vi "TagDB Refmgr-Execute Expression.vi"(8 "error in (no error)":errorcluster, 10 "expressions":cluster{"Tag":string, "formula":string}[](array[cluster]), 11 "DB Ref":T1) -> (0 "error out":errorcluster, 1 "time(ms)":u32, 3 "DB Ref (dup)":T1)   [LabVIEW 2017, in "TagDB UIStateExpression.lvlib"]
uses:
  TagDB UIStateExpression.lvlib
  <userlib>/_NEVSTOP/TagDB/Typedef/TagDB.ctl
  <userlib>/_OpenG.lib/string/string.llb/Trim Whitespace (String)__ogtk.vi
  <userlib>/_OpenG.lib/string/string.llb/Trim Whitespace (String Array)__ogtk.vi
  <userlib>/_OpenG.lib/array/array.llb/Filter 1D Array with Scalar (String)__ogtk.vi
  <userlib>/_NEVSTOP/TagDB/TagDB.lvlib
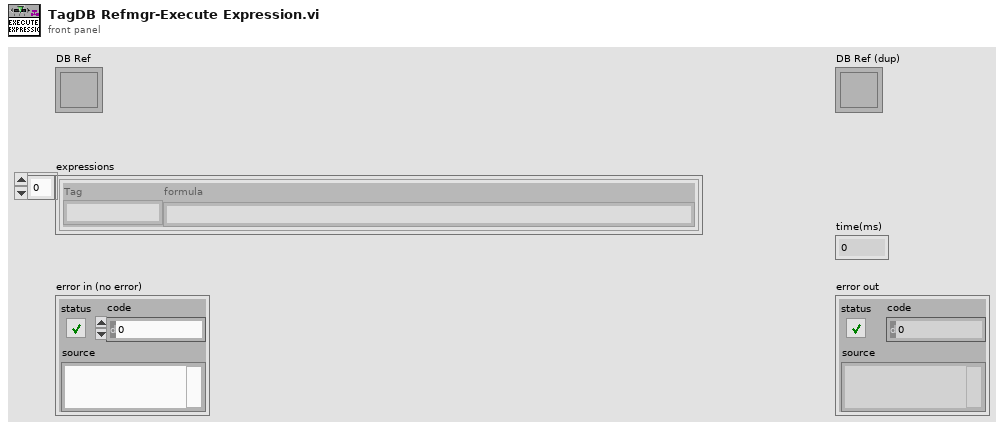
[diagram p1: front panel]
types:
  T1 = typedef "TagDB.lvlib/TagDB.ctl" = refnum<k1>
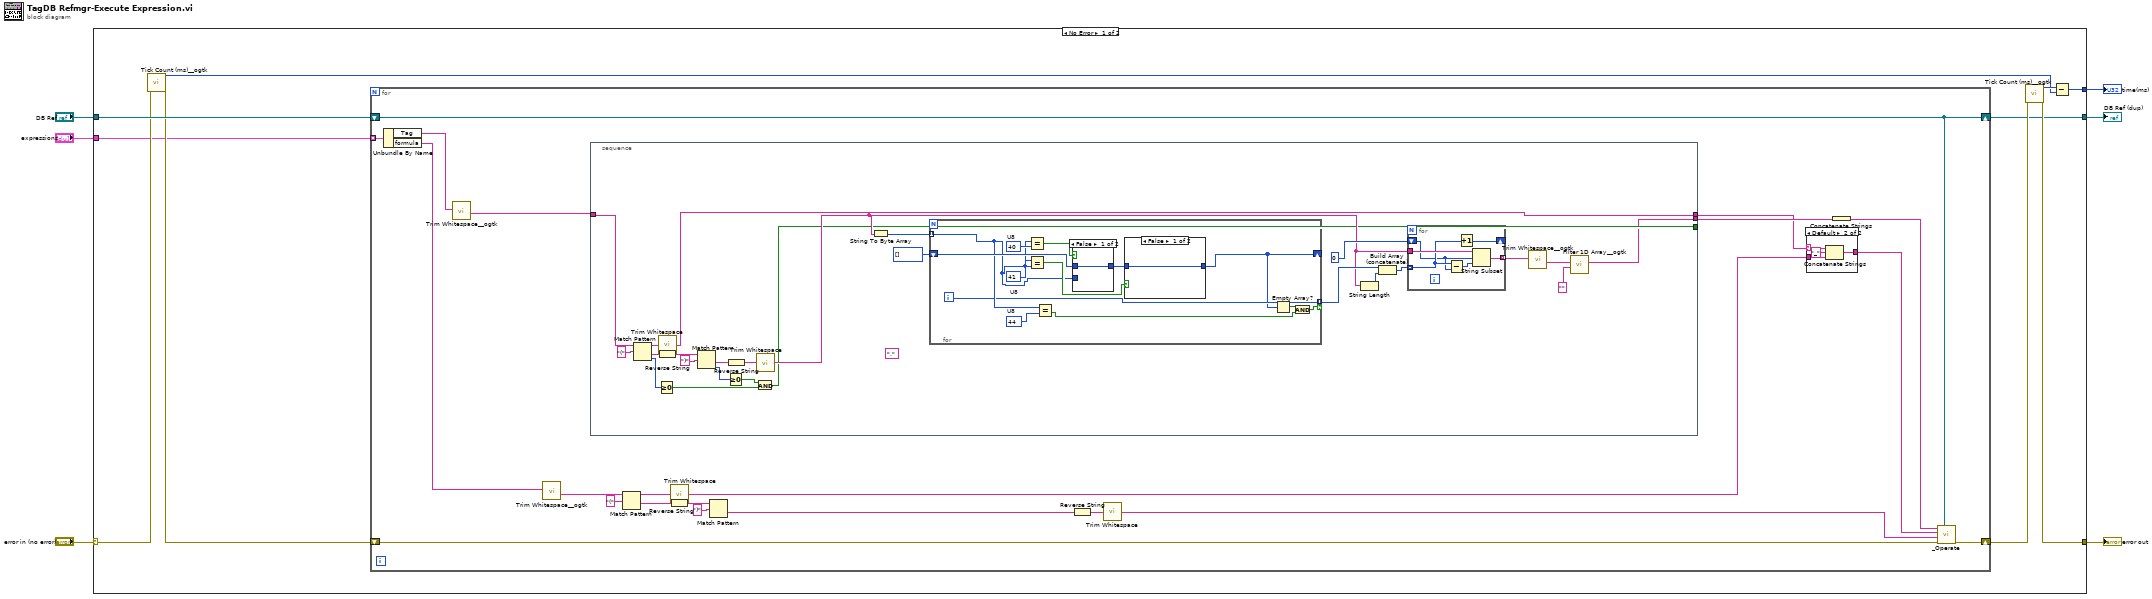
[diagram p0: block diagram]
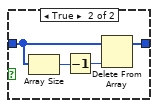
[diagram p2: hidden frame]
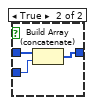
[diagram p3: hidden frame]
diagram:
  n1 = case shown="No Error" "error in (no error)" {
    selector: "error in (no error)" -> [w15 w97]
    tunnel: [w12 w97] -> w5
    tunnel: "DB Ref" -> [w16 w96]
    tunnel: [w8 w96] -> w1
    tunnel: [w9 _] -> w3
    tunnel: "expressions" -> [w7 _]
    frame No Error {
      n2 = call <userlib>:"Tick Count (ms)__ogtk.vi"("error in (no error)"=w15) -> ("error out"=w13:errorcluster, "millisecond timer value"=w10:u32)  [unwired: 9 in]
      n3 = for {
        tunnel: w7 -> [w37] mode=indexing
        shift-right: [w35] -> w14
        shift-left: w13 -> [w36]
        shift-right: [w34] -> w8
        shift-left: w16 -> [w34]
        n4 = Unbundle By Name(w37) -> ("Tag"=w33:string, "formula"=w32:string)
        n5 = call-poly <userlib>:"Trim Whitespace__ogtk.vi"("String in"=w33) -> ("String out"=w31:string)  [unwired: 6 in]
        n6 = call-poly <userlib>:"Trim Whitespace__ogtk.vi"("String in"=w32) -> ("String out"=w21:string)  [unwired: 6 in]
        n7 = stacked-sequence {
          tunnel: [w48] -> _
          tunnel: [w43] -> w30
          tunnel: [w52] -> w29
          tunnel: w31 -> [w40]
          frame #0 {
            (unwired) "," ("regular expression")
            n8 = Match Pattern(string=w40, regular expression="(") -> (before substring=w39:string, after substring=w41:string, offset past match=w44:i32)  [unwired: 1 in, 1 out]
            n9 = Greater Or Equal To 0?(x=w44) -> (x >= 0?=w47:bool)
            n10 = call <vilib>:"Trim Whitespace.vi"("string"=w39) -> ("trimmed string"=w52:string)  [unwired: 1 in]
            n11 = Reverse String(1:w41) -> (0:w49:string)
            n12 = Match Pattern(string=w49, regular expression=")") -> (after substring=w50:string, offset past match=w45:i32)  [unwired: 1 in, 2 out]
            n13 = Greater Or Equal To 0?(x=w45) -> (x >= 0?=w46:bool)
            n14 = Reverse String(1:w50) -> (0:w51:string)
            n15 = And(x=w46, y=w47) -> (x .and. y?=w48:bool)
            n16 = call <vilib>:"Trim Whitespace.vi"("string"=w51) -> ("trimmed string"=w53:string)  [unwired: 1 in]
            n17 = String To Byte Array(string=w53) -> (unsigned byte array=w55:u8[])
            n18 = for {
              tunnel: w55 -> [w74] mode=indexing
              shift-right: [w71] -> _
              shift-left: i32[] [] -> [w76]
              tunnel: [w73] -> w56 mode=indexing if=w70
              i -> [w73]
              w75 = u8 44  # U8
              w79 = u8 41  # U8
              w81 = u8 40  # U8
              n19 = Equal?(x=w74, y=w81) -> (x = y?=w80:bool)
              n20 = Equal?(x=w79, y=w74) -> (x = y?=w77:bool)
              n21 = Equal?(x=w74, y=w75) -> (x = y?=w69:bool)
              n22 = case shown="False" w80 {
                tunnel: w76 -> [w87 w90]
                tunnel: w74 -> [_ w89]
                tunnel: [w87 w88] -> w78
                frame False {
                }
                frame True {
                  n23 = Build Array (concatenate)(w90, w89) -> (w88:i32[])
                }
              }
              n24 = case shown="False" w77 {
                tunnel: w78 -> [w82 w85]
                tunnel: [w82 w83] -> w71
                frame False {
                }
                frame True {
                  n25 = Array Size(array=w85) -> (size(s)=w86:i32)
                  n26 = Decrement(x=w86) -> (x-1=w84:i32)
                  n27 = Delete From Array(array=w85, index=w84) -> (array with subset deleted=w83:i32[])  [unwired: 1 in, 1 out]
                }
              }
              n28 = Empty Array?(array=w71) -> (empty?=w72:bool)
              n29 = And(x=w72, y=w69) -> (x .and. y?=w70:bool)
            }
            n30 = String Length(string=w53) -> (length=w60:i32)
            n31 = Build Array (concatenate)(w56, w60) -> (w59:i32[])
            n32 = for {
              tunnel: w53 -> [w68]
              tunnel: w59 -> [w66] mode=indexing
              tunnel: [w67] -> w58 mode=indexing
              shift-right: [w63] -> _
              shift-left: 0 ("Numeric") -> [w64]
              n33 = Subtract(x=w66, y=w64) -> (x-y=w65:i32)
              n34 = Increment(x=w66) -> (x+1=w63:i32)
              n35 = String Subset(string=w68, offset (0)=w64, length (rest)=w65) -> (substring=w67:string)
            }
            n36 = call-poly <userlib>:"Trim Whitespace__ogtk.vi"("String in"=w58) -> ("String out"=w61:string[])  [unwired: 6 in]
            n37 = call-poly <userlib>:"Filter 1D Array__ogtk.vi"("items to filter"="" ("trimmed string"), "array"=w61) -> ("filtered array"=w43:string[])  [unwired: 4 in, 1 out]
          }
        }
        n38 = Match Pattern(string=w21, regular expression="(") -> (before substring=w27:string, after substring=w26:string)  [unwired: 1 in, 2 out]
        n39 = call <vilib>:"Trim Whitespace.vi"("string"=w27) -> ("trimmed string"=w20:string)  [unwired: 1 in]
        n40 = Reverse String(1:w26) -> (0:w24:string)
        n41 = Match Pattern(string=w24, regular expression=")") -> (after substring=w23:string)  [unwired: 1 in, 3 out]
        n42 = Reverse String(1:w23) -> (0:w22:string)
        n43 = call <vilib>:"Trim Whitespace.vi"("string"=w22) -> ("trimmed string"=w17:string)  [unwired: 1 in]
        n44 = case shown="Default" w29 {
          selector: w29 -> [_ w95]
          tunnel: w20 -> [w91 w94]
          tunnel: [w91 w93] -> w18
          frame "" {
          }
          frame Default {
            n45 = Concatenate Strings(w95, "_" ("string"), w94) -> (w93:string)
          }
        }
        n46 = Concatenate Strings(w30) -> (w19:string)
        n47 = call "_Operate.vi"("DB Ref"=w34, "error in (no error)"=w36, "parameter"=w17, "Operation"=w18, "Ctrl"=w19) -> ("error out"=w35:errorcluster)  [unwired: 6 in]
      }
      n48 = call <userlib>:"Tick Count (ms)__ogtk.vi"("error in (no error)"=w14) -> ("error out"=w12:errorcluster, "millisecond timer value"=w11:u32)  [unwired: 9 in]
      n49 = Subtract(x=w11, y=w10) -> (x-y=w9:u32)
    }
    frame Error {
    }
  }
  "error out" <- w5
  "time(ms)" <- w3
  "DB Ref (dup)" <- w1
